vi "LS372_read_only_Check_Queue.vi"(7 "error in (no error)":errorcluster, 10 "queue":refnum<queue>) -> (0 "error out":errorcluster, 1 "LS372_only_read-Cluster Control":T1, 3 "New Entries?":bool)   [LabVIEW 2019]
uses:
  LS372/LS372_read_only-Control.ctl
panel:
  out "Numeric":i32
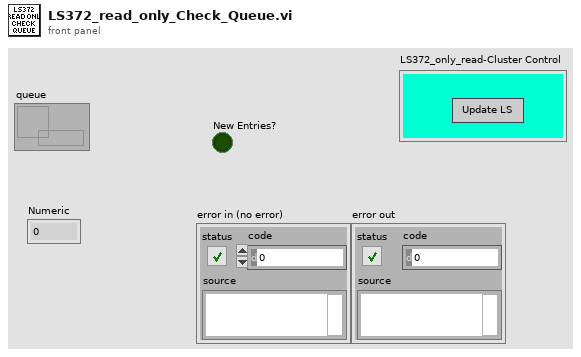
[diagram p1: front panel]
types:
  T1 = typedef "LS372_read_only-Control.ctl" = cluster{"Update Lakeshores":bool}
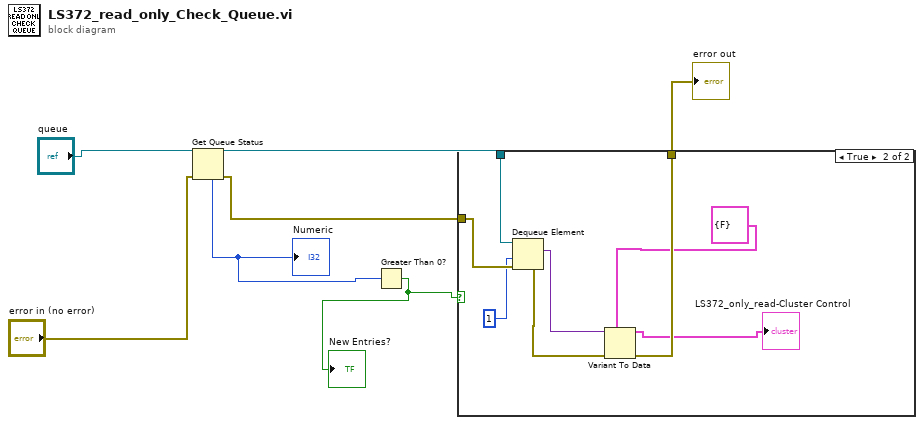
[diagram p0: block diagram]
diagram:
  n1 = Get Queue Status(queue="queue", error in (no error)="error in (no error)") -> (queue out=w6:refnum<queue>, error out=w5:errorcluster, # elements in queue=w3:i32)  [unwired: 1 in, 5 out]
  "Numeric" <- w3
  n2 = Greater Than 0?(x=w3) -> (x > 0?=w2:bool)
  "New Entries?" <- w2
  n3 = case shown="True" w2 {
    tunnel: w6 -> [_ w16]
    tunnel: w5 -> [w8 w15]
    tunnel: [w8 w11] -> w1
    frame False {
    }
    frame True {
      n4 = Dequeue Element(queue=w16, timeout in ms (-1)=1, error in (no error)=w15) -> (element=w13:variant, error out=w12:errorcluster)  [unwired: 2 out]
      n5 = Variant To Data(error in=w12, type=T1 {"Update Lakeshores"=FALSE} ("LS372_only_read-Cluster Control"), Variant=w13) -> (data=→"LS372_only_read-Cluster Control":T1, error out=w11:errorcluster)
    }
  }
  "error out" <- w1
